vi "Step DAO.vi"(8 "error in (no error)":errorcluster, 9 "Step Count In":string, 10 "Step In":T2[](array[typedef]), 11 "Step DAO Actions":T1) -> (0 "error out":errorcluster, 1 "Step Count Out":string, 2 "Step Out":T2[](array[typedef]), 3 "Start Time":timestamp, 5 "Duplicates found":bool)   [LabVIEW 2009]
uses:
  Messages/Target.ctl
  Data Access Objects/Metadata/LBCB Number.ctl
  Step DAO Actions.ctl
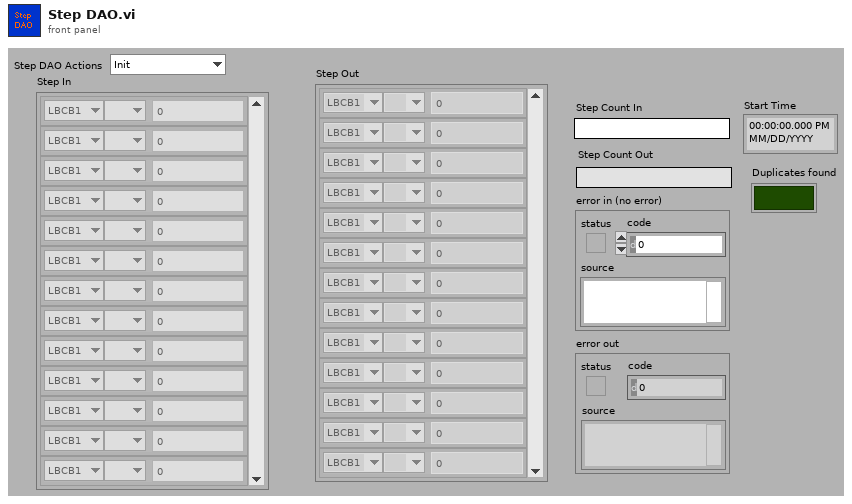
[diagram p1: front panel]
types:
  T1 = typedef "Step DAO Actions.ctl" = enum16{"Init", "Set", "Get", "Reset Count"}
  T2 = typedef "Target.ctl" = cluster{"LBCB Number":T3, "DOF Vectors":enum16{" ", "Dx", "Dy", "Dz", "Rx", "Ry", "Rz", "Fx", "Fy", "Fz", "Mx", "My", "Mz"}, "Amount":dbl}
  T3 = typedef "LBCB Number.ctl" = enum16{"LBCB1", "LBCB2"}
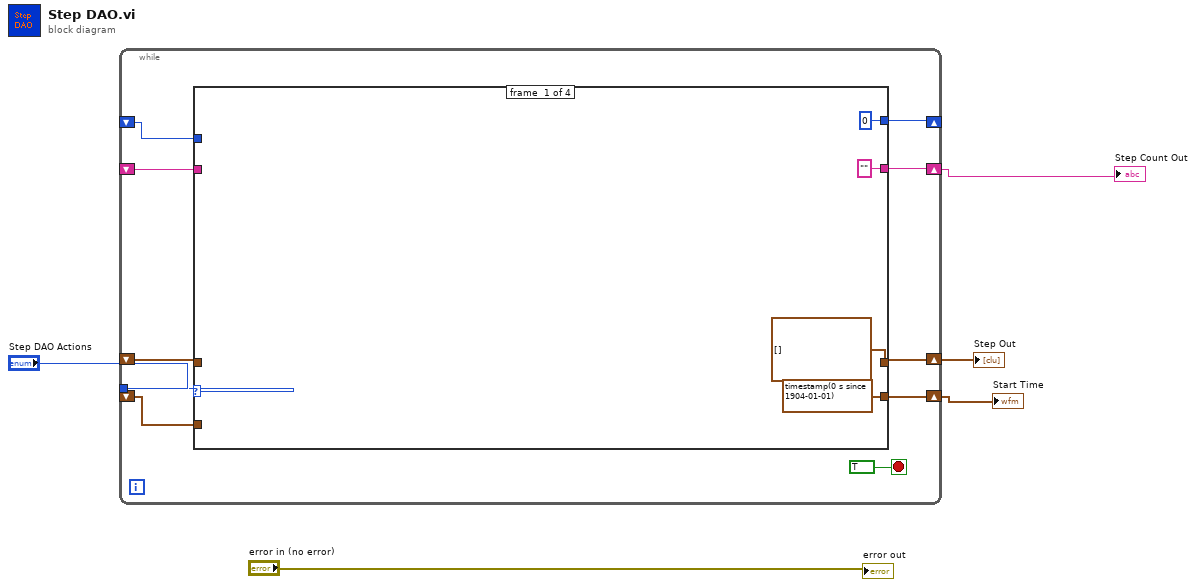
[diagram p0: block diagram]
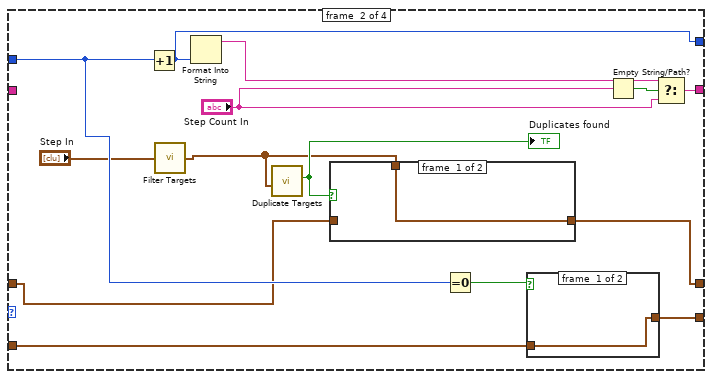
[diagram p2: hidden frame]
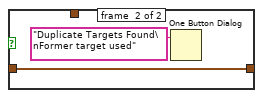
[diagram p3: hidden frame]
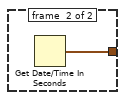
[diagram p4: hidden frame]
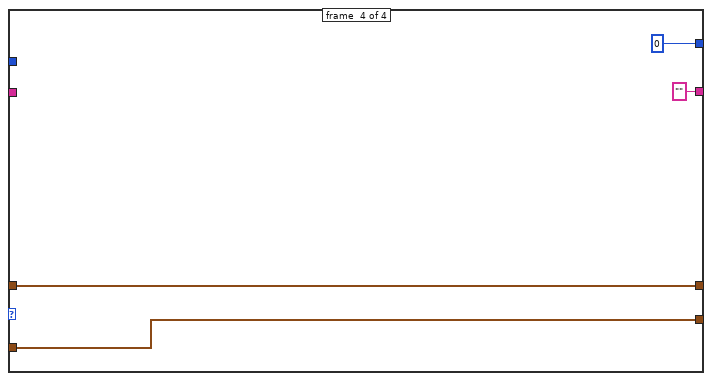
[diagram p6: hidden frame]
diagram:
  n1 = while {
    tunnel: "Step DAO Actions" -> [w14]
    shift-right: [w13] -> w4
    shift-left: _ -> [w12]
    shift-right: [w10] -> w2
    shift-left: _ -> [w8]
    shift-right: [w11] -> _
    shift-left: _ -> [w9]
    shift-right: [w7] -> w1
    shift-left: _ -> [w6]
    stop <- TRUE stop-if-true
    n2 = case shown="\"Init\"" w14 {
      tunnel: [T2[] [] ("Targets Out") w22 w42 w44] -> w13
      tunnel: w12 -> [_ w23 w42 w44]
      tunnel: [0 w25 w41 0] -> w11
      tunnel: ["" ("Step Count In") w31 w40 "" ("Step Count In")] -> w10
      tunnel: w9 -> [_ w29 w41 _]
      tunnel: w8 -> [_ _ w40 _]
      tunnel: [timestamp(0 s since 1904-01-01) ("seconds since 1Jan1904") w27 w39 w43] -> w7
      tunnel: w6 -> [_ w26 w39 w43]
      frame #0 {
      }
      frame #1 {
        n3 = Increment(x=w29) -> (x+1=w25:i32)
        n4 = call "Filter Targets.vi"("Targets In"="Step In") -> ("Targets Out"=w20:T2[])
        n5 = Format Into String(w25) -> (resulting string=w30:string)  [unwired: 3 in, 1 out]
        n6 = call "Duplicate Targets.vi"("Array"=w20) -> ("Duplicates found"=w24:bool)  [unwired: 10 out]
        "Duplicates found" <- w24
        n7 = case shown="False" w24 {
          tunnel: w23 -> [_ w36]
          tunnel: [w34 w36] -> w22
          tunnel: w20 -> [w34 _]
          frame #0 {
          }
          frame #1 {
            n8 = One Button Dialog(message="Duplicate Targets Found\nFormer target used") -> ()  [unwired: 2 out]
          }
        }
        n9 = Equal To 0?(x=w29) -> (x = 0?=w28:bool)
        n10 = case shown="False" w28 {
          tunnel: [w37 w38] -> w27
          tunnel: w26 -> [w37 _]
          frame #0 {
          }
          frame #1 {
            n11 = Get Date/Time In Seconds() -> (seconds since 1Jan1904=w38:timestamp)
          }
        }
        n12 = Empty String/Path?(string/path="Step Count In") -> (empty?=w33:bool)
        n13 = Select(t=w30, s=w33, f="Step Count In") -> (s? t:f=w31:string)
      }
      frame #2 {
      }
      frame #3 {
      }
    }
  }
  "Step Out" <- w4
  "Step Count Out" <- w2
  "Start Time" <- w1
  "error out" <- "error in (no error)"
